vi "execute.vi"(8 "error in (no error)":errorcluster, 10 "ComponentData.lvclass":refnum<class "ComponentData.lvclass">, 11 "ReadyState in":refnum<class "EnabledState.lvclass">) -> (0 "error out":errorcluster, 2 "ComponentData.lvclass 2":refnum<class "ComponentData.lvclass">, 3 "ReadyState out":refnum<class "EnabledState.lvclass">)   [LabVIEW 2013, in "ComponentData.lvlib" / "EnabledState.lvclass"]
uses:
  <userlib>/Common/Component/Application/RT/ComponentData/ComponentState/EnabledState/EnabledState.lvclass
  <userlib>/Common/Component/Application/RT/ComponentData/ComponentData/ComponentData.lvclass
  <userlib>/Common/Component/Application/RT/ComponentData/ComponentState/ComponentState/ComponentState.lvclass
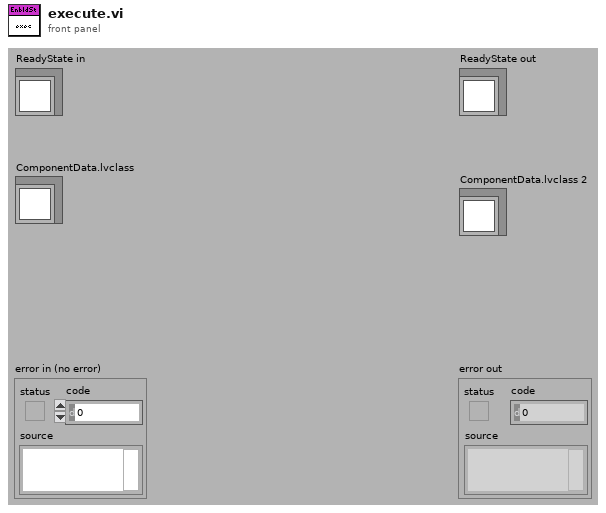
[diagram p1: front panel]
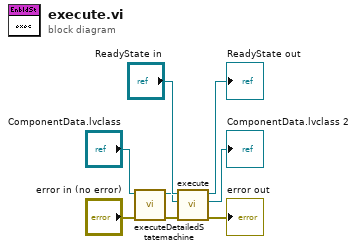
[diagram p0: block diagram]
diagram:
  n1 = call-dynamic "executeDetailedStatemachine.vi"("error in (no error)"="error in (no error)", "ComponentData in"="ComponentData.lvclass") -> ("error out"=w2:errorcluster, "ComponentData out"=w1:refnum<class "ComponentData.lvclass">)  [unwired: 8 in]
  n2 = call-parent "execute.vi"("error in (no error)"=w2, "ComponentData.lvclass"=w1, "ComponentState in"="ReadyState in") -> ("error out"=→"error out":errorcluster, "ComponentData.lvclass 2"=→"ComponentData.lvclass 2":refnum<class "ComponentData.lvclass">, "ComponentState out"=→"ReadyState out":refnum<class "EnabledState.lvclass">)  [unwired: 6 in]
